vi "Instrument_check.vi"(0 "VISA resource in":refnum<visa-resource-name>) -> (1 "VISA resource out":refnum<visa-resource-name>, 2 "Response":string, 3 "Status":bool)   [LabVIEW 2017]
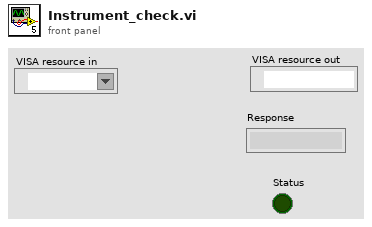
[diagram p1: front panel]
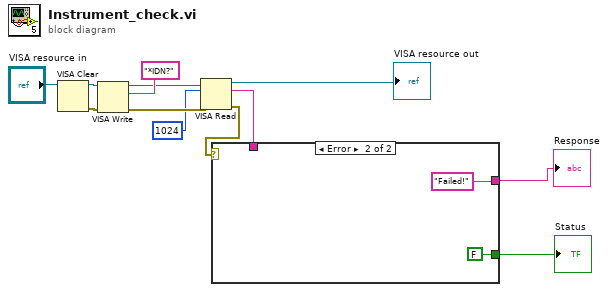
[diagram p0: block diagram]
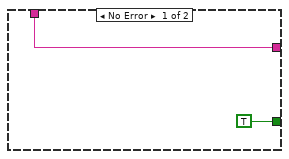
[diagram p2: hidden frame]
diagram:
  n1 = VISA Clear(VISA resource name="VISA resource in") -> (VISA resource name out=w11:refnum<visa-resource-name>, error out=w10:errorcluster)  [unwired: 1 in]
  n2 = VISA Write(VISA resource name=w11, write buffer="*IDN?", error in (no error)=w10) -> (VISA resource name out=w8:refnum<visa-resource-name>, error out=w7:errorcluster)  [unwired: 1 out]
  n3 = VISA Read(VISA resource name=w8, byte count=u32 1024, error in (no error)=w7) -> (VISA resource name out=→"VISA resource out":refnum<visa-resource-name>, read buffer=w3:string, error out=w4:errorcluster)  [unwired: 1 out]
  n4 = case shown="Error" w4 {
    tunnel: [w14 "Failed!"] -> w5
    tunnel: w3 -> [w14 _]
    tunnel: [TRUE ("Status") FALSE ("Status")] -> w2
    frame No Error {
    }
    frame Error {
    }
  }
  "Response" <- w5
  "Status" <- w2
